vi "Load New Measurement.vi"(8 "error in (no error)":errorcluster, 11 "UI in":refnum<class "Controller UI.lvclass">) -> (0 "error out":errorcluster, 3 "UI out":refnum<class "Controller UI.lvclass">)   [LabVIEW 2016, in "Controller UI.lvlib" / "Controller UI.lvclass"]
uses:
  <userlib>/Common Components/Controller UI/Controller UI.lvclass
  C:/Program Files (x86)/National Instruments/LabVIEW 2016/vi.lib/ActorFramework/Actor/Actor.lvclass
  <vilib>/ActorFramework/Actor/Actor.lvclass/Actor.ctl
  <userlib>/Common Components/Controller/Messages/Load Measurements/Find Measurements On Disk Message.lvclass
  <userlib>/Common Components/Controller/Messages/Populate Mesaurements in UI/Display Measurements Message.lvclass
  <vilib>/ActorFramework/Actor/Actor.lvclass
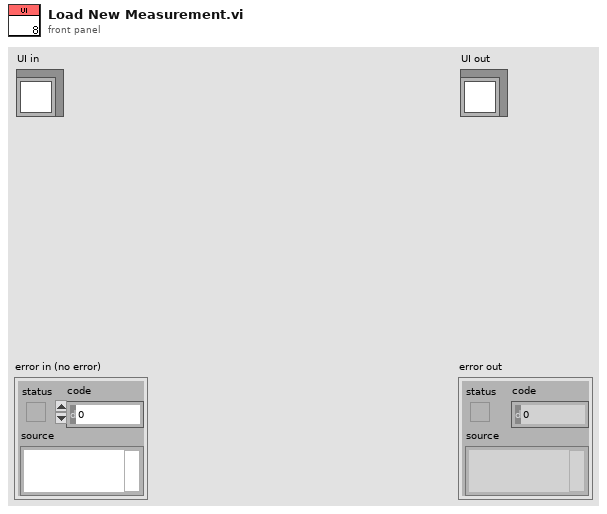
[diagram p1: front panel]
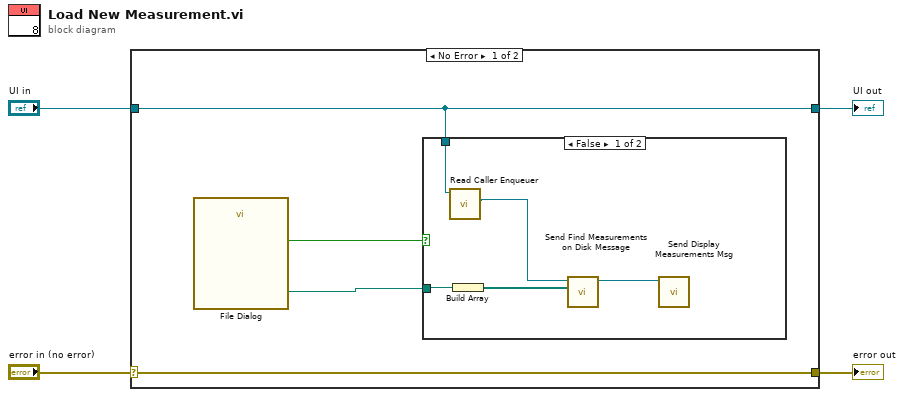
[diagram p0: block diagram]
diagram:
  n1 = case shown="No Error" "error in (no error)" {
    selector: "error in (no error)" -> [w8 w15]
    tunnel: [w8 w15] -> w3
    tunnel: [w5 w14] -> w1
    tunnel: "UI in" -> [w5 w14]
    frame No Error {
      n2 = call "File Dialog"() -> ("selected path"=w7:path, "cancelled"=w6:bool)  [unwired: 12 in, 2 out]
      n3 = case shown="False" w6 {
        tunnel: w7 -> [w10 _]
        tunnel: w5 -> [w12 _]
        frame False {
          n4 = call <vilib>:"Read Caller Enqueuer.vi"("Actor"=w12) -> ("Caller Enqueuer"=w11:refnum<class "Message Enqueuer.lvclass">)  [unwired: 10 in]
          n5 = Build Array(w10) -> (w9:path[])
          n6 = call <userlib>:"Send Find Measurements on Disk Message.vi"("Measurement Locations"=w9, "Message Enqueuer in"=w11) -> ("Message Enqueuer out"=w13:refnum<class "Message Enqueuer.lvclass">)  [unwired: 8 in, 1 out]
          n7 = call <userlib>:"Send Display Measurements Msg.vi"("Message Enqueuer in"=w13) -> ()  [unwired: 9 in, 2 out]
        }
        frame True {
        }
      }
    }
    frame Error {
    }
  }
  "error out" <- w3
  "UI out" <- w1
